vi "OFDM-SIM添加CP.vi"(1 "输入符号":cdb[](array[numeric])) -> (0 "加CP后":cdb[](array[numeric]))   [LabVIEW 2018]
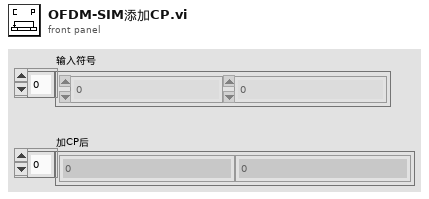
[diagram p1: front panel]
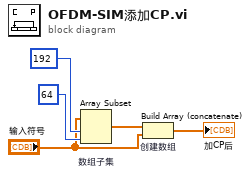
[diagram p0: block diagram]
diagram:
  n1 = Array Subset "数组子集"(array="输入符号", index=192 ("索引"), length=64 ("长度")) -> (w3:cdb[])
  n2 = Build Array (concatenate) "创建数组"(w3, "输入符号") -> (→"加CP后":cdb[])
